vi "Scanner.vi"() -> ()   [LabVIEW 2012]
uses:
  Database.lvclass
  Image.lvclass
panel:
  out "iDatabase":i32
  in  "y corrector":dbl=1.0
  in  "x corrector":dbl=1.0
  out "Vessel Cluster":T1
  out "Scan Clusters":T2(array[cluster])
  out "Image":T3(plugin-control)
  in  "Scan Properties":T4={"X Size"=512.0, "Y Size"=512.0, "lens"=20.0, "mag"=1.0}
  in  "condition":string
  in  "stop":bool
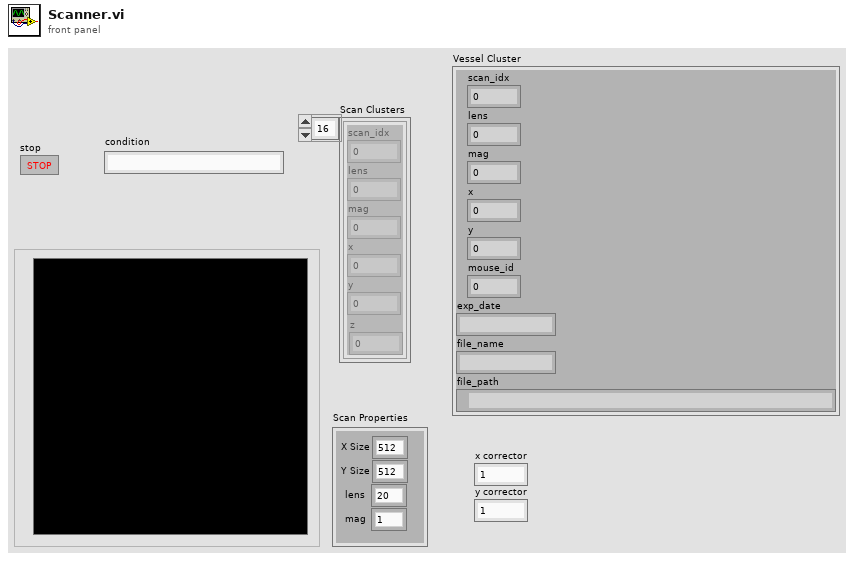
[diagram p1: front panel]
types:
  T1 = cluster{"scan_idx":i32, "lens":i32, "mag":dbl, "x":dbl, "y":dbl, "mouse_id":i32, "exp_date":string, "file_name":string, "file_path":path}
  T2 = cluster{"scan_idx":dbl, "lens":dbl, "mag":dbl, "x":dbl, "y":dbl, "z":dbl}[]
  T3 = typedef "IMAQ Image.ctl" = refnum<image>
  T4 = cluster{"X Size":dbl, "Y Size":dbl, "lens":dbl, "mag":dbl}
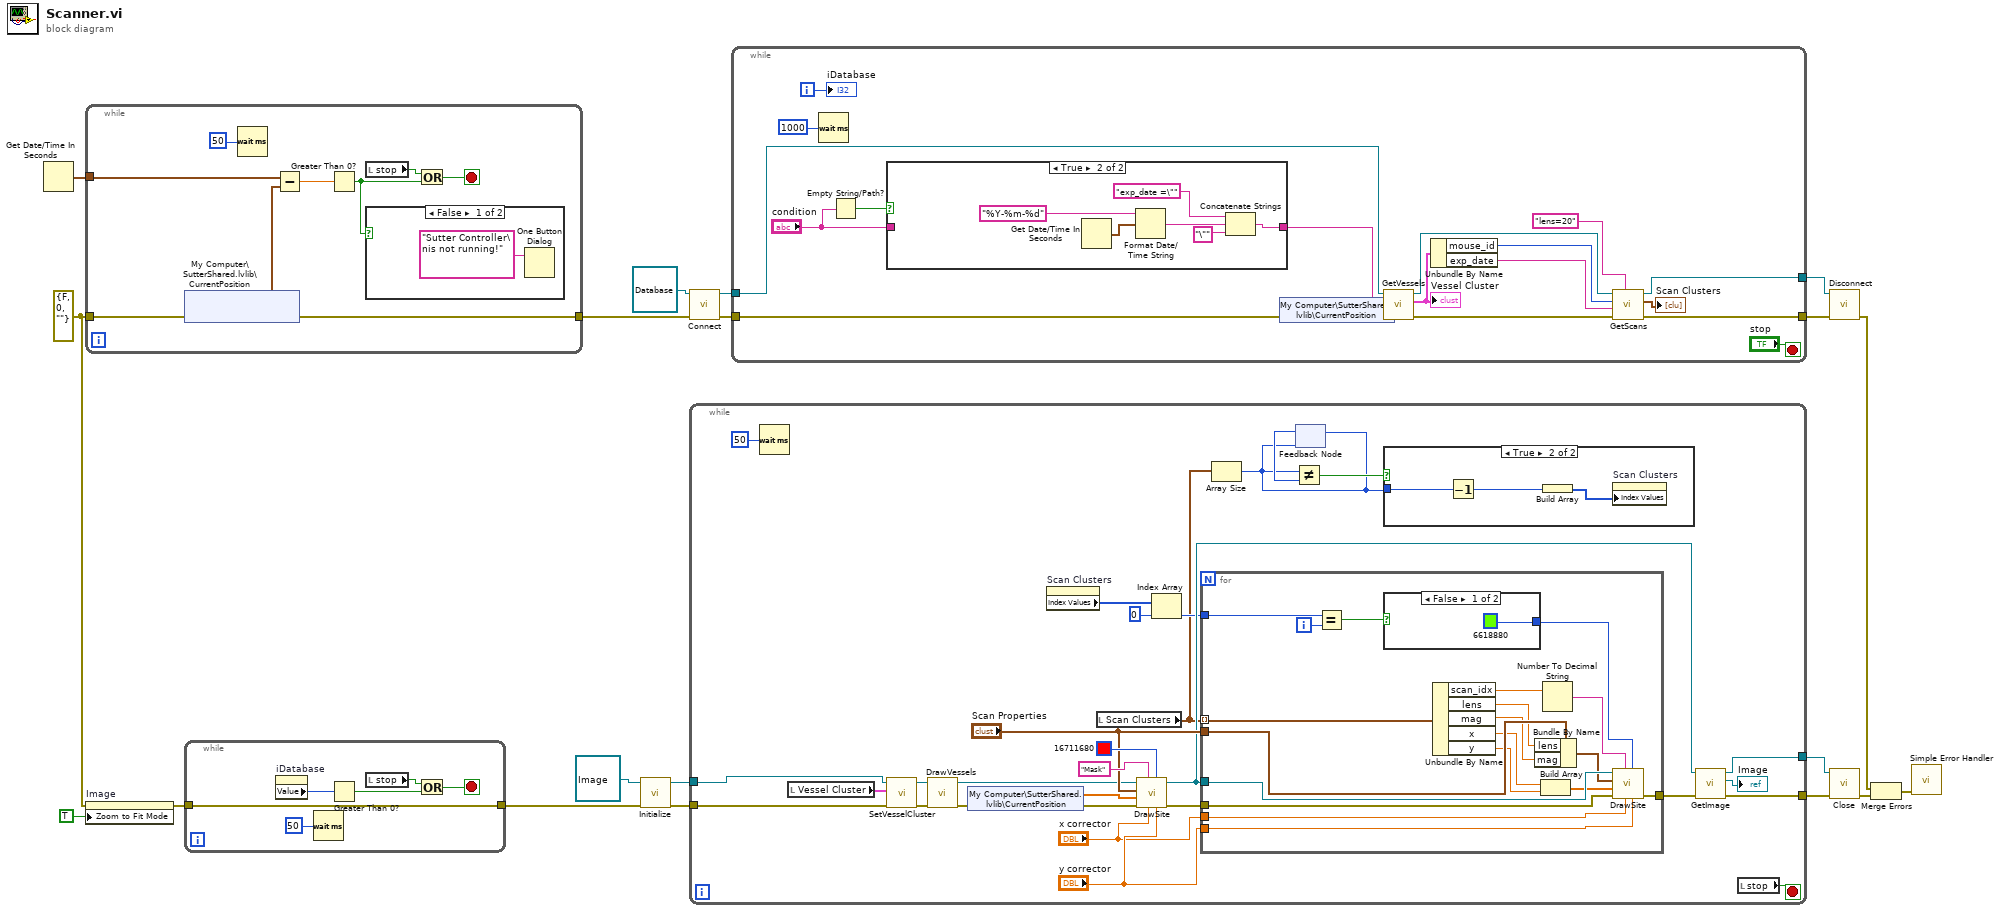
[diagram p0: block diagram]
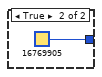
[diagram p4: hidden frame]
diagram:
  w4 = errorcluster {"status"=FALSE, "code"=0, "source"=""} ("error in (no error)")
  n1 = Get Date/Time In Seconds() -> (seconds since 1Jan1904=w1:timestamp)
  n2 = while {
    tunnel: w4 -> [w25]
    tunnel: [w24] -> w3
    tunnel: w1 -> [w22]
    stop <- w27 stop-if-true
    n3 = shared-variable "My Computer\\SutterShared.lvlib\\CurrentPosition"(error in=w25) -> (error out=w24:errorcluster, w23:timestamp)  [unwired: 1 out]
    n4 = Wait (ms)(milliseconds to wait=u32 50) -> ()  [unwired: 1 out]
    n5 = Subtract(x=w22, y=w23) -> (x-y=w21:dbl)
    n6 = Greater Than 0?(x=w21) -> (x > 0?=w20:bool)
    n7 = local read "stop"() -> (w26:bool)
    n8 = case shown="False" w20 {
      frame False {
        n9 = One Button Dialog(message="Sutter Controller\nis not running!") -> ()  [unwired: 1 in, 1 out]
      }
      frame True {
      }
    }
    n10 = Or(x=w26, y=w20) -> (x .or. y?=w27:bool)
  }
  n11 = property on="Image" class="ImageControl"(error in=w4, "Zoom to Fit Mode"=TRUE) -> (error out=w6:errorcluster)  [unwired: 1 in, 1 out]
  n12 = while {
    tunnel: w6 -> [w33]
    tunnel: [w33] -> w5
    stop <- w30 stop-if-true
    n13 = property on="iDatabase" class="DigNum (strict)"() -> ("Value"=w35:i32)  [unwired: 2 in, 2 out]
    n14 = Wait (ms)(milliseconds to wait=u32 50) -> ()  [unwired: 1 out]
    n15 = Greater Than 0?(x=w35) -> (x > 0?=w32:bool)
    n16 = local read "stop"() -> (w31:bool)
    n17 = Or(x=w31, y=w32) -> (x .or. y?=w30:bool)
  }
  n18 = call-dynamic "Initialize.vi"("error in (no error)"=w5, "Image in"=refnum<class "Image.lvclass"> refnum) -> ("error out"=w9:errorcluster, "Image out"=w10:refnum<class "Image.lvclass">)  [unwired: 8 in]
  n19 = call-dynamic "Connect.vi"("error in (no error)"=w3, "Database in"=refnum<class "Database.lvclass"> refnum) -> ("error out"=w16:errorcluster, "Database out"=w19:refnum<class "Database.lvclass">)  [unwired: 8 in]
  n20 = while {
    tunnel: w10 -> [w63]
    tunnel: w9 -> [w62]
    tunnel: [w61] -> w8
    tunnel: [w60] -> w7
    stop <- w64 stop-if-true
    n21 = Wait (ms)(milliseconds to wait=u32 50) -> ()  [unwired: 1 out]
    n22 = local read "Vessel Cluster"() -> (w53:T1)
    n23 = call-dynamic "SetVesselCluster.vi"("error in (no error)"=w62, "Vessel Cluster"=w53, "Image in"=w63) -> ("error out"=w52:errorcluster, "Image out"=w59:refnum<class "Image.lvclass">)  [unwired: 7 in]
    n24 = call-dynamic "DrawVessels.vi"("error in (no error)"=w52, "Image in"=w59) -> ("error out"=w37:errorcluster, "Image out"=w51:refnum<class "Image.lvclass">)  [unwired: 8 in]
    n25 = shared-variable "My Computer\\SutterShared.lvlib\\CurrentPosition"(error in=w37) -> (w38:dbl[], error out=w36:errorcluster)
    n26 = property on="Scan Clusters" class="Arr (strict)"() -> ("Index Values"=w45:u32[])  [unwired: 2 in, 2 out]
    n27 = local read "Scan Clusters"() -> (w42:T2)
    n28 = call-dynamic "DrawSite.vi"("y corrector"="y corrector", "Color"=u32 16711680, "x corrector"="x corrector", "Group"="Mask", "error in (no error)"=w36, "Position"=w38, "Scan Properties"="Scan Properties", "Image in"=w51) -> ("error out"=w49:errorcluster, "Image out"=w50:refnum<class "Image.lvclass">)  [unwired: 2 in]
    n29 = Index Array(array=w45, index=0) -> (element=w43:u32)
    n30 = for {
      tunnel: w50 -> [w86]
      tunnel: w42 -> [w84] mode=indexing
      tunnel: "Scan Properties" -> [w83]
      tunnel: w49 -> [w75]
      tunnel: [w74] -> w48
      tunnel: "y corrector" -> [w73]
      tunnel: "x corrector" -> [w72]
      tunnel: w43 -> [w70]
      i -> [w71]
      n31 = Equal?(x=w70, y=w71) -> (x = y?=w69:bool)
      n32 = case shown="False" w69 {
        tunnel: [u32 6618880 ("Color") u32 16769905 ("Color")] -> w68
        frame False {
        }
        frame True {
        }
      }
      n33 = Unbundle By Name(w84) -> ("scan_idx"=w78:dbl, "lens"=w77:dbl, "mag"=w76:dbl, "x"=w81:dbl, "y"=w80:dbl)
      n34 = Bundle By Name(cluster=w83, "lens"=w77, "mag"=w76) -> (w82:T4)
      n35 = Build Array(w81, w80) -> (w79:dbl[])
      n36 = Number To Decimal String(number=w78) -> (decimal integer string=w85:string)  [unwired: 1 in]
      n37 = call-dynamic "DrawSite.vi"("y corrector"=w73, "Color"=w68, "x corrector"=w72, "Group"=w85, "error in (no error)"=w75, "Position"=w79, "Scan Properties"=w82, "Image in"=w86) -> ("error out"=w74:errorcluster)  [unwired: 2 in, 1 out]
    }
    n38 = Array Size(array=w42) -> (size(s)=w39:i32)
    n39 = feedback-in #1(w39) -> ()
    n40 = feedback #1(w39) -> (w41:i32)
    n41 = Not Equal?(x=w39, y=w41) -> (x != y?=w40:bool)
    n42 = case shown="True" w40 {
      tunnel: w39 -> [_ w66]
      frame False {
      }
      frame True {
        n43 = Decrement(x=w66) -> (x-1=w65:i32)
        n44 = Build Array(w65) -> (w67:i32[])
        n45 = property on="Scan Clusters" class="Arr (strict)"("Index Values"=w67) -> ()  [unwired: 2 in, 2 out]
      }
    }
    n46 = call-dynamic "GetImage.vi"("error in (no error)"=w48, "Image in"=w50) -> ("error out"=w60:errorcluster, "Image"=→"Image":T3, "Image out"=w61:refnum<class "Image.lvclass">)  [unwired: 7 in]
    n47 = local read "stop"() -> (w64:bool)
  }
  n48 = while {
    tunnel: w19 -> [w107]
    tunnel: [w106] -> w17
    tunnel: w16 -> [w92]
    tunnel: [w105] -> w15
    i -> [w93]
    stop <- "stop" stop-if-true
    n49 = Wait (ms)(milliseconds to wait=u32 1000) -> ()  [unwired: 1 out]
    n50 = Empty String/Path?(string/path="condition") -> (empty?=w103:bool)
    n51 = case shown="True" w103 {
      tunnel: [w108 w112] -> w101
      tunnel: "condition" -> [w108 _]
      frame False {
      }
      frame True {
        n52 = Get Date/Time In Seconds() -> (seconds since 1Jan1904=w111:timestamp)
        n53 = Format Date/Time String(time format string (%c)="%Y-%m-%d", seconds (now)=w111) -> (date/time string=w109:string)  [unwired: 1 in]
        n54 = Concatenate Strings("exp_date =\"", w109, "\"" ("string")) -> (w112:string)
      }
    }
    n55 = shared-variable "My Computer\\SutterShared.lvlib\\CurrentPosition"(error in=w92) -> (w90:dbl[], error out=w91:errorcluster)
    n56 = call-dynamic "GetVessels.vi"("error in (no error)"=w91, "Position"=w90, "condition"=w101, "Database in"=w107) -> ("error out"=w99:errorcluster, "Vessel Cluster"=w96:T1, "Database out"=w100:refnum<class "Database.lvclass">)  [unwired: 5 in]
    "Vessel Cluster" <- w96
    n57 = Unbundle By Name(w96) -> ("mouse_id"=w98:i32, "exp_date"=w97:string)
    n58 = call-dynamic "GetScans.vi"("condition"="lens=20", "error in (no error)"=w99, "exp_date"=w97, "mouse_id"=w98, "Database in"=w100) -> ("error out"=w105:errorcluster, "Scan Clusters"=→"Scan Clusters":T2, "Database out"=w106:refnum<class "Database.lvclass">)  [unwired: 4 in]
    "iDatabase" <- w93
  }
  n59 = call-dynamic "Disconnect.vi"("error in (no error)"=w15, "Database in"=w17) -> ("error out"=w2:errorcluster)  [unwired: 8 in, 1 out]
  n60 = call-dynamic "Close.vi"("error in (no error)"=w7, "Image in"=w8) -> ("error out"=w13:errorcluster)  [unwired: 8 in, 1 out]
  n61 = Merge Errors(w2, w13) -> (w12:errorcluster)
  n62 = call <vilib>:"Simple Error Handler.vi"("error in (no error)"=w12) -> ()  [unwired: 4 in, 5 out]
